vi "Drive_Encoder.vi"() -> ()   [LabVIEW 2012]
uses:
  Robot Global Data.vi
panel:
  out "error out":errorcluster
  out "Current angleR (deg)":dbl(knob) scale=0.0..360.0
  out "DistanceR (in)":dbl
  out "RevolutionsR":dbl
  out "EncoderR Rate (deg/sec)":dbl
  in  "Reset EncoderR?":bool
  out "EncoderR Alarm Status":string
  out "EncoderR Direction":string
  out "EncoderL Direction":string
  out "EncoderL Alarm Status":string
  in  "Reset EncoderL?":bool
  out "EncoderL Rate (deg/sec)":dbl
  out "RevolutionsL":dbl
  out "DistanceL (in)":dbl
  out "Current angleL (deg)":dbl(knob) scale=0.0..360.0
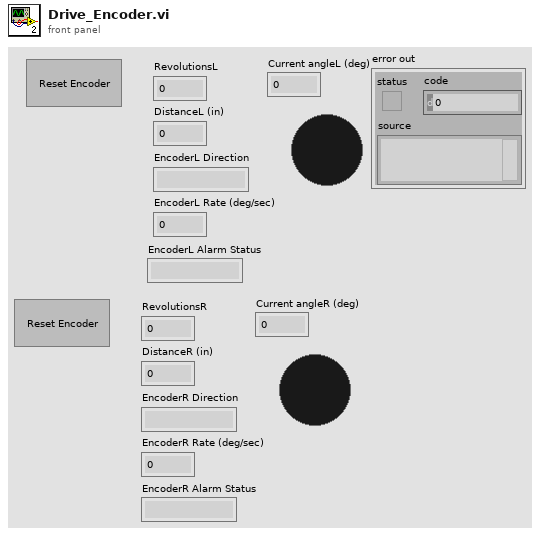
[diagram p1: front panel]
types:
  T1 = typedef "WPI_EncoderDevRef.ctl" = cluster{"DevStatus":errorcluster, "EncoderIndex":T2, "CounterIndex":T3, "DistancePerCount":dbl, "Decoding Type":T4}
  T2 = typedef "FPGA_EncoderIdx.ctl" = enum8{"Enc 0", "Enc 1", "Enc 2", "Enc 3", "Invalid"}
  T3 = typedef "FPGA_CounterCtrSystemIndex.ctl" = enum8{"Ctr 0", "Ctr 1", "Ctr 2", "Ctr 3", "Ctr 4", "Ctr 5", "Ctr 6", "Ctr 7", "Invalid"}
  T4 = typedef "WPI_EncoderType.ctl" = enum16{"1x", "2x", "4x"}
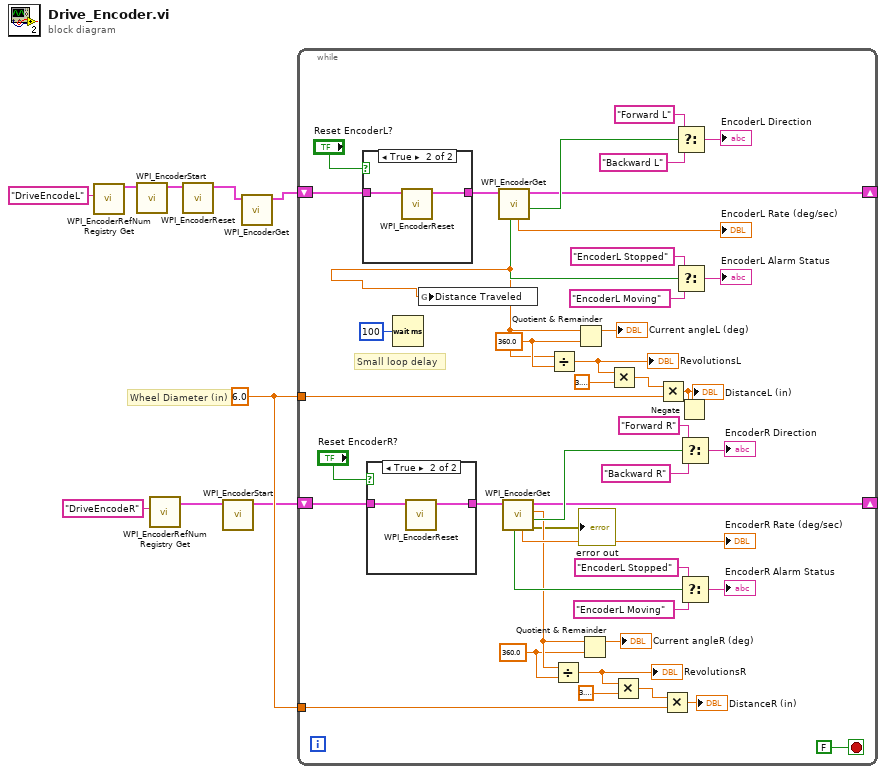
[diagram p0: block diagram]
diagram:
  w7 = 6.0 ("y")
  # "Wheel Diameter (in)"
  n1 = call <vilib>:"WPI_EncoderRefNum Registry Get.vi"("refnum name"="DriveEncodeL") -> ("EncoderDevRef"=w9:T1)  [unwired: 9 in, 1 out]
  n2 = call <vilib>:"WPI_EncoderStart.vi"("EncoderDevRef"=w9) -> ("EncoderDevRef"=w3:T1)  [unwired: 1 in, 9 out]
  n3 = call <vilib>:"WPI_EncoderRefNum Registry Get.vi"("refnum name"="DriveEncodeR") -> ("EncoderDevRef"=w6:T1)  [unwired: 9 in, 1 out]
  n4 = call <vilib>:"WPI_EncoderReset.vi"("EncoderDevRef"=w3) -> ("EncoderDevRef"=w2:T1)  [unwired: 1 in, 9 out]
  n5 = call <vilib>:"WPI_EncoderStart.vi"("EncoderDevRef"=w6) -> ("EncoderDevRef"=w4:T1)  [unwired: 1 in, 9 out]
  n6 = call <vilib>:"WPI_EncoderGet.vi"("EncoderDevRef"=w2) -> ("EncoderDevRef"=w1:T1)  [unwired: 1 in, 9 out]
  n7 = while {
    shift-right: [w47] -> _
    shift-left: w1 -> [w52]
    tunnel: w7 -> [w35]
    tunnel: w7 -> [w16]
    shift-right: [w14] -> _
    shift-left: w4 -> [w15]
    stop <- FALSE stop-if-true
    w21 = 360.0 ("y")
    w40 = 360.0 ("y")
    # "Small loop delay"
    n8 = case shown="True" "Reset EncoderL?" {
      tunnel: w52 -> [w58 w60]
      tunnel: [w58 w59] -> w50
      frame False {
      }
      frame True {
        n9 = call <vilib>:"WPI_EncoderReset.vi"("EncoderDevRef"=w60) -> ("EncoderDevRef"=w59:T1)  [unwired: 1 in, 9 out]
      }
    }
    n10 = case shown="True" "Reset EncoderR?" {
      tunnel: w15 -> [w55 w57]
      tunnel: [w55 w56] -> w31
      frame False {
      }
      frame True {
        n11 = call <vilib>:"WPI_EncoderReset.vi"("EncoderDevRef"=w57) -> ("EncoderDevRef"=w56:T1)  [unwired: 1 in, 9 out]
      }
    }
    n12 = Wait (ms)(milliseconds to wait=u32 100) -> ()  [unwired: 1 out]
    n13 = call <vilib>:"WPI_EncoderGet.vi"("EncoderDevRef"=w50) -> ("Direction"=w49:bool, "Distance"=w10:dbl, "EncoderDevRef"=w47:T1, "Rate"=→"EncoderL Rate (deg/sec)":dbl, "Stopped"=w48:bool)  [unwired: 1 in, 5 out]
    n14 = global write "Robot Global Data.vi" "Distance Traveled"(w10) -> ()
    n15 = call <vilib>:"WPI_EncoderGet.vi"("EncoderDevRef"=w31) -> ("error out"=→"error out":errorcluster, "Direction"=w30:bool, "Distance"=w22:dbl, "EncoderDevRef"=w14:T1, "Rate"=→"EncoderR Rate (deg/sec)":dbl, "Stopped"=w29:bool)  [unwired: 1 in, 4 out]
    n16 = Divide(x=w10, y=w40) -> (x/y=w39:dbl)
    "RevolutionsL" <- w39
    n17 = Divide(x=w22, y=w21) -> (x/y=w20:dbl)
    "RevolutionsR" <- w20
    n18 = Quotient & Remainder(x=w10, y=w40) -> (x-y*floor(x/y)=→"Current angleL (deg)":dbl)  [unwired: 1 out]
    n19 = Quotient & Remainder(x=w22, y=w21) -> (x-y*floor(x/y)=→"Current angleR (deg)":dbl)  [unwired: 1 out]
    n20 = Multiply(x=w39, y=3.141592653589793) -> (x*y=w37:dbl)
    n21 = Multiply(x=w20, y=3.141592653589793) -> (x*y=w18:dbl)
    n22 = Multiply(x=w37, y=w35) -> (x*y=w11:dbl)
    "DistanceL (in)" <- w11
    n23 = Multiply(x=w18, y=w16) -> (x*y=→"DistanceR (in)":dbl)
    n24 = Select(t="Forward L", s=w49, f="Backward L") -> (s? t:f=→"EncoderL Direction":string)
    n25 = Select(t="EncoderL Stopped", s=w48, f="EncoderL Moving") -> (s? t:f=→"EncoderL Alarm Status":string)
    n26 = Negate(x=w11) -> ()  [unwired: 1 out]
    n27 = Select(t="Forward R", s=w30, f="Backward R") -> (s? t:f=→"EncoderR Direction":string)
    n28 = Select(t="EncoderL Stopped", s=w29, f="EncoderL Moving") -> (s? t:f=→"EncoderR Alarm Status":string)
  }
